vi "fpga_status.vi"(8 "error in (no error)":errorcluster, 11 "USRP_1_x_200MHz in":refnum<class "USRP_1_x_200MHz.lvclass">) -> (0 "error out":errorcluster, 2 "pulse TX status":T1, 3 "USRP_1_x_200MHz out":refnum<class "USRP_1_x_200MHz.lvclass">)   [LabVIEW 2021, in "USRP_1_x_200MHz.lvclass"]
uses:
  USRP_1_x_200MHz.lvclass
  USRP_1_x_200MHz.lvclass/USRP_1_x_200MHz.ctl
  <vilib>/rvi/interface/nirviReadWriteControl/nirviReadWriteControl.xnode
  NiFpgaLv.dll
  <vilib>/Utility/error.llb/Error Cluster From Error Code.vi
  <vilib>/rvi/interface/Simulation/niFpgaSimulationCallBeginRW.vi
  <vilib>/rvi/errors/niLvFpgaAdjustHostInterfaceError.vi
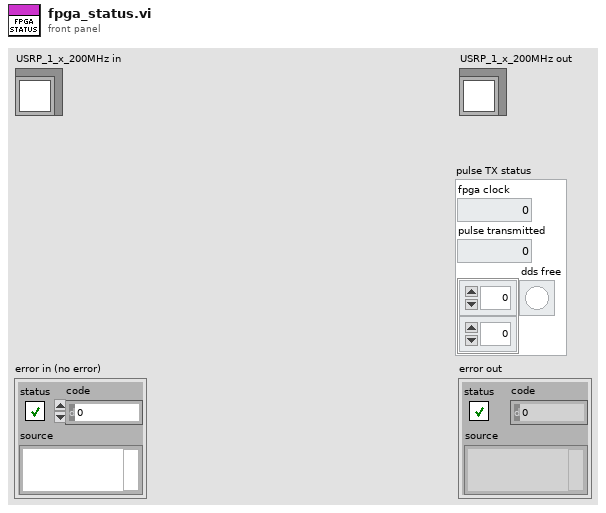
[diagram p1: front panel]
types:
  T1 = cluster{"fpga clock":dbl, "pulse transmitted":u32, "dds free":bool[][]}
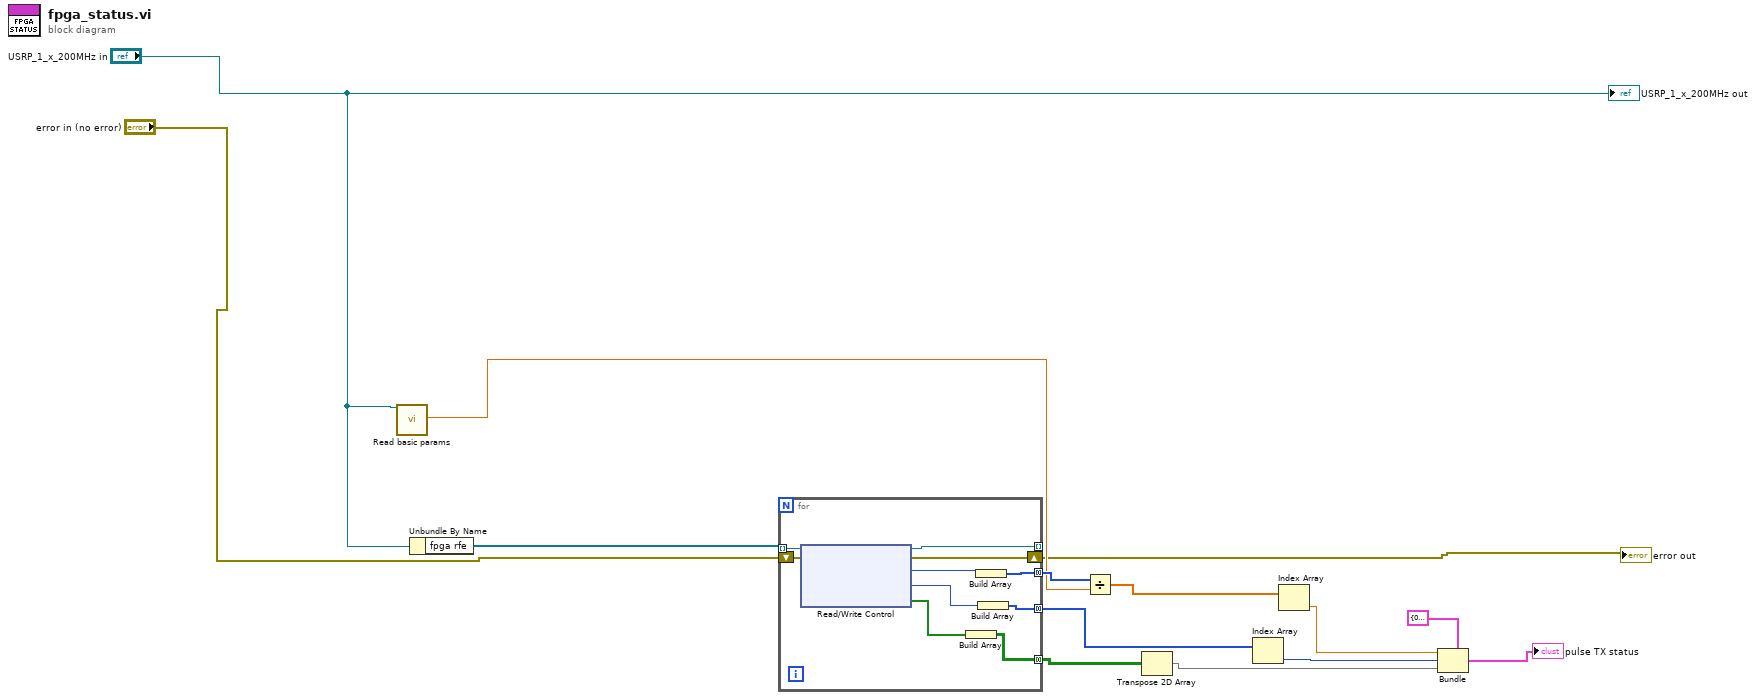
[diagram p0: block diagram]
diagram:
  n1 = call-dynamic "Read basic params.vi"("device_type in"="USRP_1_x_200MHz in") -> ("Fs  FPGA"=w11:dbl)  [unwired: 13 in, 5 out]
  n2 = Unbundle By Name("USRP_1_x_200MHz in") -> ("fpga rfe"=w13:refnum<k20>[])
  n3 = for {
    tunnel: w13 -> [w21] mode=indexing
    shift-right: [w23] -> w3
    shift-left: "error in (no error)" -> [w24]
    tunnel: [w22] -> _ mode=indexing
    tunnel: [w19] -> w12 mode=concatenating
    tunnel: [w17] -> w6 mode=concatenating
    tunnel: [w15] -> w14 mode=concatenating
    n4 = xnode "Read/Write Control"("FPGA VI Reference In"=w21, "error in"=w24) -> ("FPGA VI Reference Out"=w22:refnum<k20>, "error out"=w23:errorcluster, "fpga clock"=w16:u64, "pulse transmitted"=w18:u32, "tx free"=w20:bool[])
    n5 = Build Array(w20) -> (w19:bool[][])
    n6 = Build Array(w16) -> (w15:u64[])
    n7 = Build Array(w18) -> (w17:u32[])
  }
  "error out" <- w3
  n8 = Divide(x=w14, y=w11) -> (x/y=w8:dbl[])
  n9 = Transpose 2D Array(2D array=w12) -> (transposed array=w9:bool[][])
  n10 = Index Array(array=w6) -> (element=w5:u32)  [unwired: 1 in]
  n11 = Index Array(array=w8) -> (element=w7:dbl)  [unwired: 1 in]
  n12 = Bundle(cluster=T1 {"fpga clock"=0.0, "pulse transmitted"=0, "dds free"=[[FALSE, FALSE, FALSE, FALSE, FALSE, FALSE, FALSE, FALSE, FALSE, FALSE, FALSE, FALSE, FALSE, FALSE, FALSE, FALSE]]} ("pulse TX status"), "fpga clock"=w7, "pulse transmitted"=w5, "dds free"=w9) -> (→"pulse TX status":T1)
  "USRP_1_x_200MHz out" <- "USRP_1_x_200MHz in"
